vi "GV_Bypass_Main.vi"() -> ()   [LabVIEW 2019]
uses:
  GV_Bypass_Global.vi
panel:
  out "V0":dbl
  out "Status Code":i32 format="%x"
  in  "set_m001":bool
  in  "set_p001":bool
  in  "pressure_preset":T1(ring) caption="Presets"
  out "move_pre":i32 caption="Prev. move"
  out "status_ac":u32(colorbox) caption="Status"
  out "P_now":dbl caption="Fridge pressure" format="%.2f"
  in  "P_set":dbl=10.0 caption="Set Point" format="%.2f"
  in  "enable_auto_ctrl":bool caption="Auto Control\nwith Pressure"
  in  "set_m010":bool
  in  "set_m005":bool
  in  "set_p010":bool
  in  "set_p005":bool
  out "turn_now":dbl=-0.0 caption="turns" format="%.3f"
  out "step_rel_pre":i32 caption="Prev. steps"
  out "step_corr":i32
  in  "backlash_corr":bool=TRUE caption="Backlash Correction"
  in  "calib_zero":bool
  out "step_new":i32 caption="steps"
  in  "do_full_open":bool
  in  "do_full_close":bool
  in  "sp_turn":dbl caption="Set point:" min=-0.1 max=0.3 step=0.001 format="%.3f"
  out "Status":bool=TRUE
  out "Chart":waveform(dbl)[](graph)=[{"t0"=timestamp(3783179446.718648 s since 1904-01-01), "dt"=1.0, "Y"=[-0.0], "attributes"=variant("NI_ChannelName"=variant(string "Turn"))}, {"t0"=timestamp(3783179446.718648 s since 1904-01-01), "dt"=1.0, "Y"=[0.0], "attributes"=variant("NI_ChannelName"=variant(string "Step"))}, {"t0"=timestamp(3783179446.718648 s since 1904-01-01), "dt"=1.0, "Y"=[1.298], "attributes"=variant("NI_ChannelName"=variant(string "Analog"))}]
  out "Last Measurement":timestamp=timestamp(3783179446.718648 s since 1904-01-01) format="%<%Y-%m-%d %H:%M:%S>T"
  in  "Interval":i32=1000
  out "Open":bool
  out "Close":bool
  in  "MotorStop":bool
  in  "MotorEN":bool
  out "Alarm Code":i32 format="%x"
  in  "Alarm Reset":bool
  out "Analog":dbl=1.298
  in  "CLOSE Steps":i32=100
  out "step_now":i32 caption="steps"
  in  "OPEN Steps":i32=100
  in  "VISA":refnum<visa-resource-name>="COM13"
  in  "OPEN":bool
  in  "CLOSE":bool
  in  "stop":bool
  # "Gate-Valve Bypass Control"
  # "Gear ratio = 1:32.\nAnalog range = ?...?."
  # "ms"
  # "Absolute Moves"
  # "±0.001"
  # "turns"
  # "Present Position"
  # "Limit Switches"
  # "Relative Moves (Expert Only)"
  # "Torr"
  # "Fully Closed   = 0      turns =         0 steps\nFully Opened = 0.25 turns = -1600 steps"
  # "Torr"
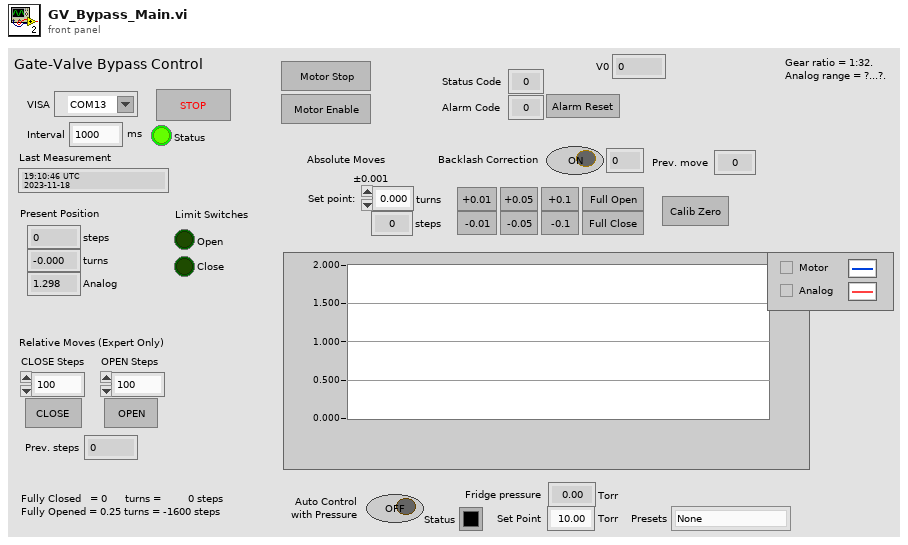
[diagram p1: front panel]
types:
  T1 = enum16{"None", "8.46 Torr  ->  1.7 K", "23.48 Torr  ->  2.0 K", "76.73 Torr  ->  2.5 K", "180.40 Torr  ->  3.0 K"}
  T2 = enum16{"None", "8.5 Torr  ->  1.7 K", "23.5 Torr  ->  2.0 K", "76.7 Torr  ->  2.5 K", "180.4 Torr  ->  3.0 K", ""}
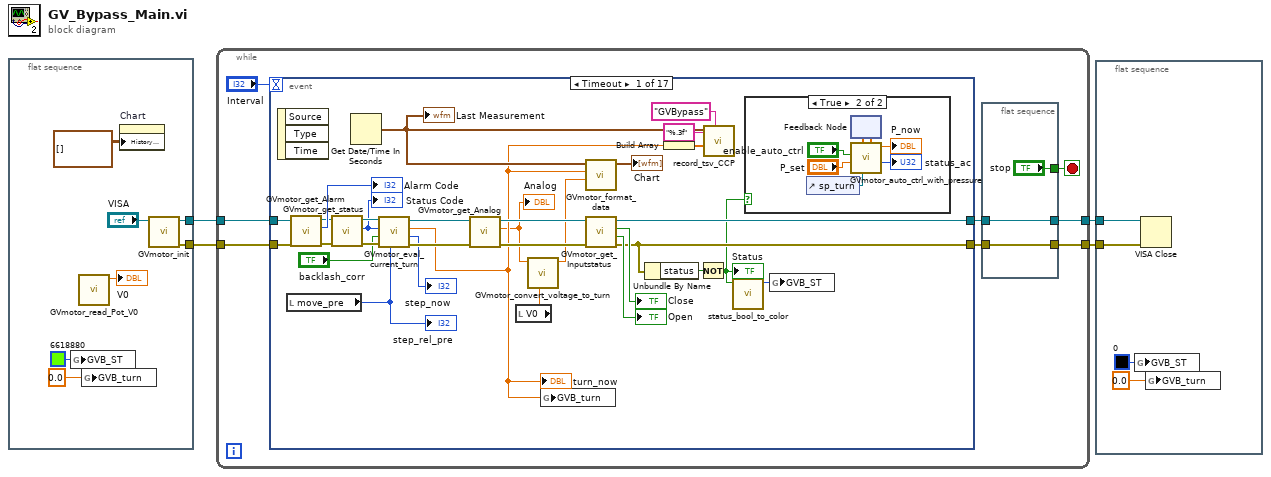
[diagram p0: block diagram]
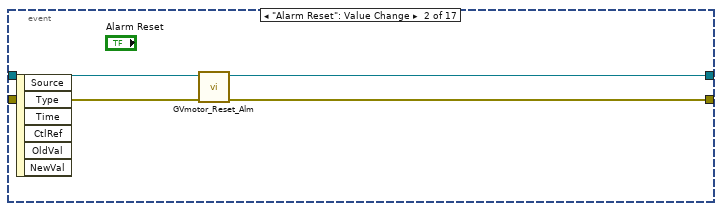
[diagram p3: hidden frame]
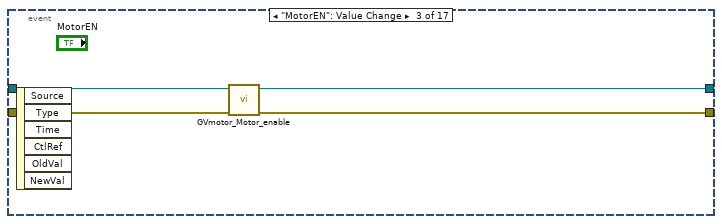
[diagram p4: hidden frame]
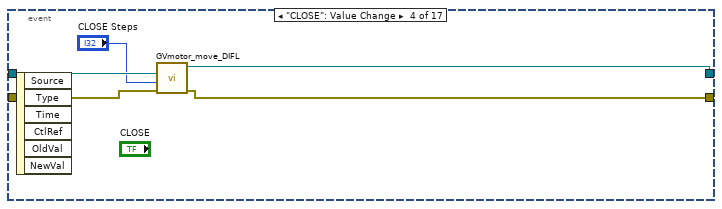
[diagram p5: hidden frame]
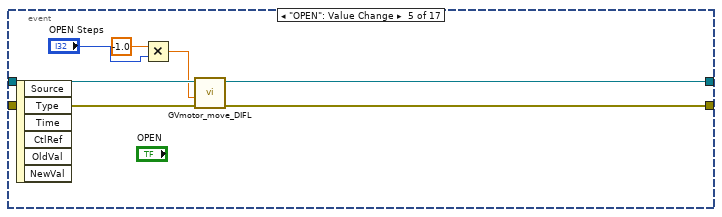
[diagram p6: hidden frame]
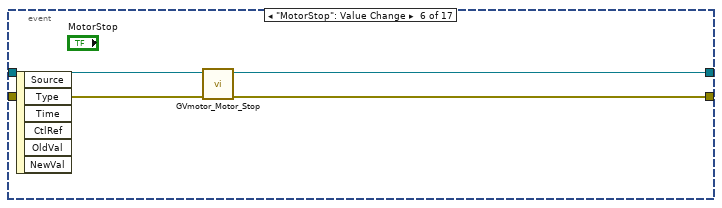
[diagram p7: hidden frame]
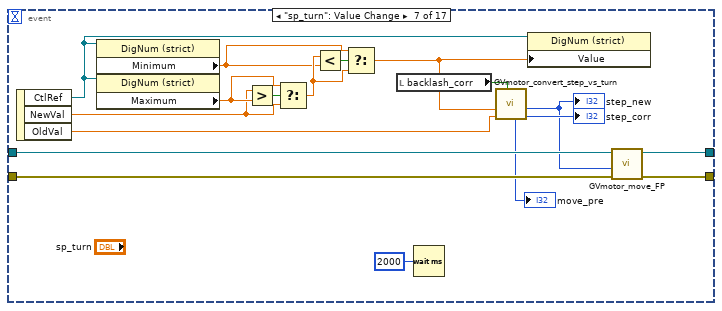
[diagram p8: hidden frame]
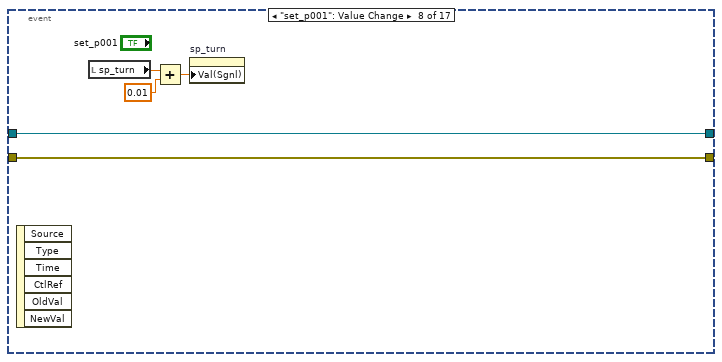
[diagram p9: hidden frame]
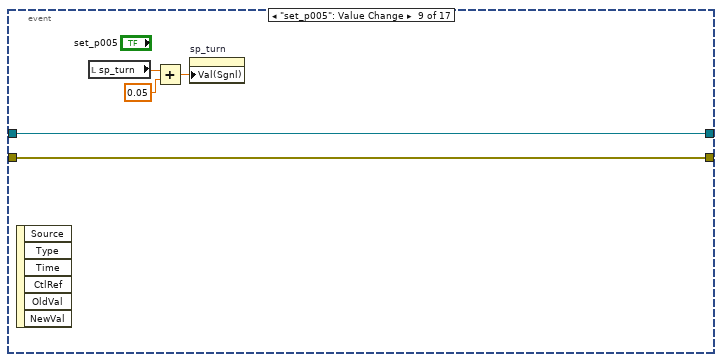
[diagram p10: hidden frame]
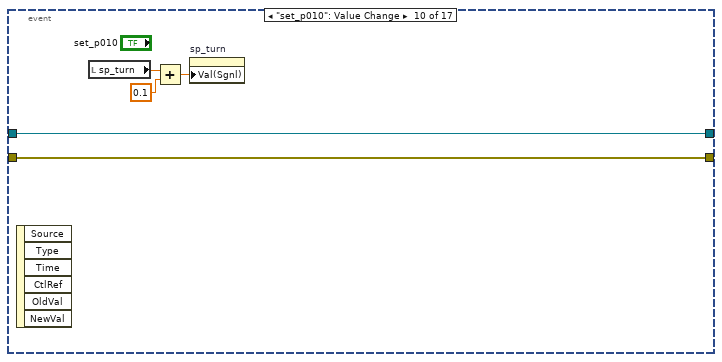
[diagram p11: hidden frame]
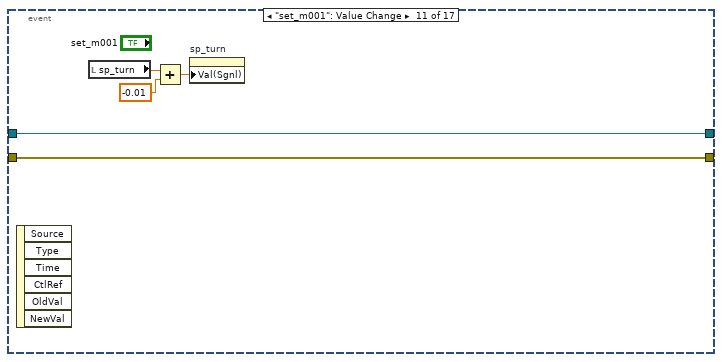
[diagram p12: hidden frame]
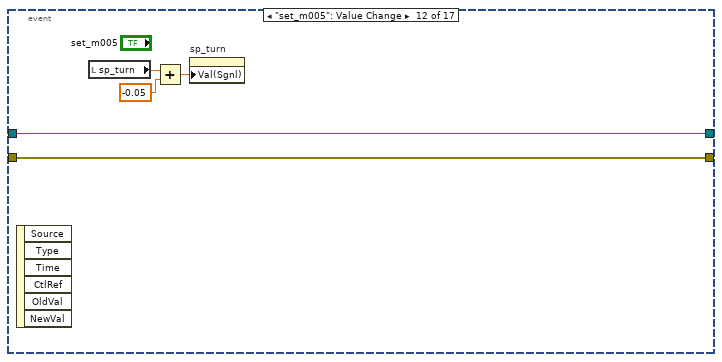
[diagram p13: hidden frame]
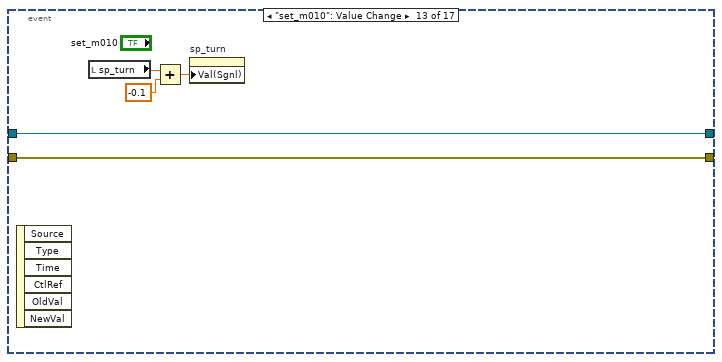
[diagram p14: hidden frame]
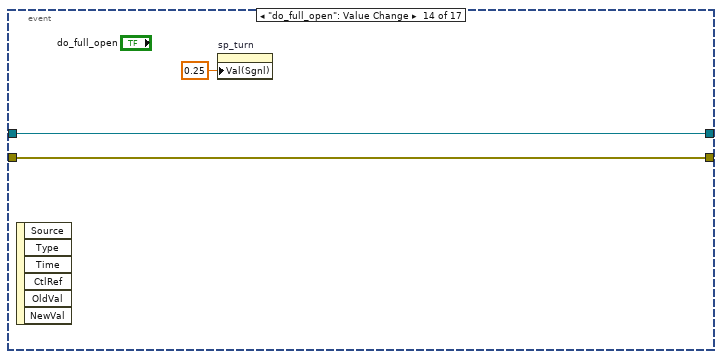
[diagram p15: hidden frame]
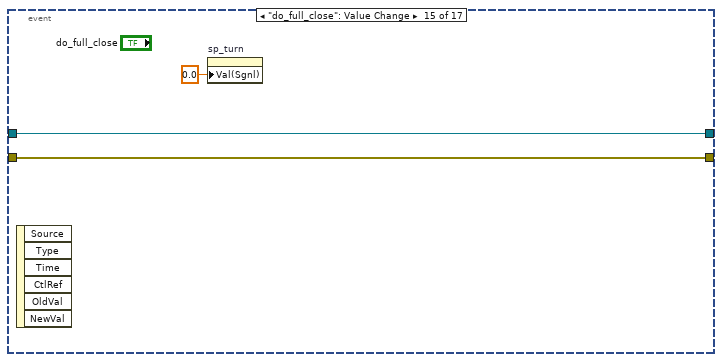
[diagram p16: hidden frame]
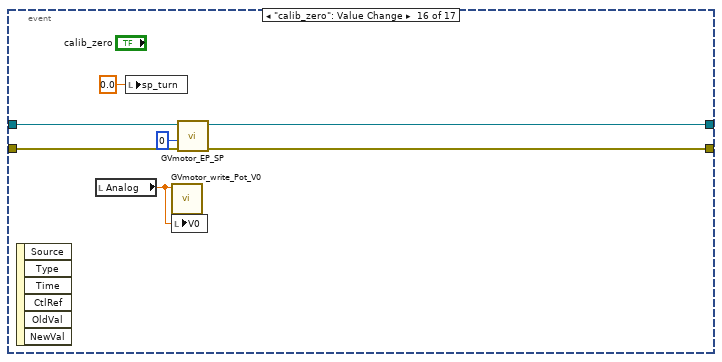
[diagram p17: hidden frame]
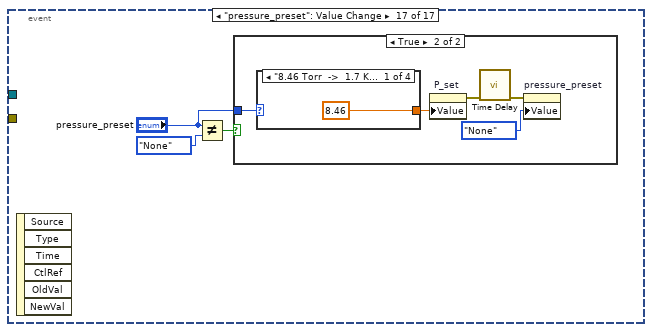
[diagram p18: hidden frame]
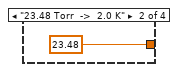
[diagram p20: hidden frame]
diagram:
  n1 = flat-sequence {
    tunnel: [w10] -> w4
    tunnel: [w9] -> w3
    frame #0 {
      n2 = global write "GV_Bypass_Global.vi" "GVB_ST"(u32 6618880 ("GVB_ST")) -> ()
      n3 = call "GVmotor_read_Pot_V0.vi"() -> ("V0"=→"V0":dbl)  [unwired: 11 in]
      n4 = global write "GV_Bypass_Global.vi" "GVB_turn"(0.0 ("GVB_opening")) -> ()
      n5 = property on="Chart" class="WFChart (strict)"("History Data"=waveform(dbl)[][] []) -> ()  [unwired: 2 in, 2 out]
      n6 = call "GVmotor_init.vi"("mWMotor_Port"="VISA") -> ("error out"=w9:errorcluster, "reference out"=w10:refnum<visa-resource-name>)  [unwired: 9 in]
    }
  }
  n7 = while {
    tunnel: w4 -> [w17]
    tunnel: w3 -> [w16]
    tunnel: [w12] -> w2
    tunnel: [w14] -> w1
    stop <- w19 stop-if-true
    n8 = event shown="[0] Timeout" {
      selector: _ -> [_ _ _ _ _ _ _ _ _ _ _ _ _ _ _ _ _]
      dyn-events: _ -> [_ _ _ _ _ _ _ _ _ _ _ _ _ _ _ _ _]
      timeout: "Interval" -> [_ _ _ _ _ _ _ _ _ _ _ _ _ _ _ _ _]
      tunnel: w17 -> [w37 w62 w65 w73 w80 w81 w87 w107 w112 w117 w122 w127 w132 w134 w137 w145 _]
      tunnel: w16 -> [w36 w63 w68 w72 w79 w84 w88 w106 w111 w116 w121 w126 w131 w133 w136 w143 _]
      tunnel: [w45 w64 w67 w71 w78 w83 w89 w106 w111 w116 w121 w126 w131 w133 w136 w142 _] -> w13
      tunnel: [w46 w61 w66 w70 w77 w82 w90 w107 w112 w117 w122 w127 w132 w134 w137 w144 _] -> w15
      event Timeout {
        n9 = event-data() -> ()  [unwired: 1 in, 3 out]
        n10 = local read "move_pre"() -> (w27:i32)
        "step_rel_pre" <- w27
        n11 = call "GVmotor_get_Alarm.vi"("error in (no error)"=w36, "VISA resource name"=w37) -> ("error out"=w35:errorcluster, "Alarm Code"=→"Alarm Code":i32, "VISA resource name out"=w34:refnum<visa-resource-name>)  [unwired: 7 in]
        n12 = call "GVmotor_get_status.vi"("error in"=w35, "VISA in"=w34) -> ("error out"=w32:errorcluster, "Status Code"=w29:i32, "VISA out"=w33:refnum<visa-resource-name>)  [unwired: 7 in]
        "Status Code" <- w29
        n13 = Get Date/Time In Seconds() -> (seconds since 1Jan1904=w42:timestamp)
        "Last Measurement" <- w42
        n14 = call "GVmotor_eval_current_turn.vi"("move_pre_sign"=w27, "error in"=w32, "backlash_corr"="backlash_corr", "status_code"=w29, "VISA in"=w33) -> ("error out"=w47:errorcluster, "step_curr"=→"step_now":i32, "turn_curr"=w26:dbl, "VISA out"=w48:refnum<visa-resource-name>)  [unwired: 3 in]
        "turn_now" <- w26
        n15 = call "GVmotor_get_Analog.vi"("error in (no error)"=w47, "VISA resource name"=w48) -> ("error out"=w30:errorcluster, "Analog"=w25:dbl, "VISA resource name out"=w31:refnum<visa-resource-name>)  [unwired: 7 in]
        "Analog" <- w25
        n16 = local read "V0"() -> (w23:dbl)
        n17 = call "GVmotor_convert_voltage_to_turn.vi"("v0"=w23, "voltage"=w25) -> ("turn"=w24:dbl)  [unwired: 8 in, 1 out]
        n18 = global write "GV_Bypass_Global.vi" "GVB_turn"(w26) -> ()
        n19 = call "GVmotor_format_data.vi"("analog"=w24, "turn"=w26, "time"=w42) -> ("waveform_array"=→"Chart":waveform(dbl)[])  [unwired: 8 in]
        n20 = call "GVmotor_get_Inputstatus.vi"("error in (no error)"=w30, "VISA resource name"=w31) -> ("error out"=w45:errorcluster, "Open"=→"Open":bool, "Close"=→"Close":bool, "VISA resource name out"=w46:refnum<visa-resource-name>)  [unwired: 6 in]
        n21 = Unbundle By Name(w45) -> ("status"=w50:bool)
        n22 = Build Array(w26) -> (w43:dbl[])
        n23 = Not(x=w50) -> (.not. x?=w39:bool)
        "Status" <- w39
        n24 = call "record_tsv_CCP.vi"("folder_name"="GVBypass", "value_array"=w43, "format"="%.3f", "time"=w42) -> ()  [unwired: 6 in, 2 out]
        n25 = call "status_bool_to_color.vi"("status_bool_1"=w39) -> ("status_color"=w49:u32)  [unwired: 10 in]
        n26 = case shown="True" w39 {
          frame False {
          }
          frame True {
            n27 = control-ref of="sp_turn"() -> (w54:refnum<vi>)
            n28 = feedback #1() -> (w59:dbl[])  [unwired: 1 in]
            n29 = call "GVmotor_auto_ctrl_with_pressure.vi"("ref_turn_set"=w54, "array_value_in"=w59, "P_set"="P_set", "enable_auto_ctrl"="enable_auto_ctrl") -> ("auto_ctrl_status"=→"status_ac":u32, "P_now"=→"P_now":dbl, "array_value_out"=w60:dbl[])  [unwired: 4 in, 1 out]
            n30 = feedback-in #1(w60) -> ()
          }
        }
        n31 = global write "GV_Bypass_Global.vi" "GVB_ST"(w49) -> ()
      }
      event "Alarm Reset": Value Change {
        n32 = event-data() -> ()  [unwired: 1 in, 6 out]
        n33 = call "GVmotor_Reset_Alm.vi"("error in (no error)"=w63, "VISA resource name"=w62) -> ("error out"=w64:errorcluster, "VISA resource name out"=w61:refnum<visa-resource-name>)  [unwired: 8 in]
      }
      event "MotorEN": Value Change {
        n34 = event-data() -> ()  [unwired: 1 in, 6 out]
        n35 = call "GVmotor_Motor_enable.vi"("error in (no error)"=w68, "VISA resource name"=w65) -> ("error out"=w67:errorcluster, "VISA resource name out"=w66:refnum<visa-resource-name>)  [unwired: 8 in]
      }
      event "CLOSE": Value Change {
        n36 = event-data() -> ()  [unwired: 1 in, 6 out]
        n37 = call "GVmotor_move_DIFL.vi"("error in"=w72, "relative_step"="CLOSE Steps", "VISA in"=w73) -> ("error out"=w71:errorcluster, "VISA out"=w70:refnum<visa-resource-name>)  [unwired: 7 in]
      }
      event "OPEN": Value Change {
        n38 = event-data() -> ()  [unwired: 1 in, 6 out]
        n39 = Multiply(x=-1.0, y="OPEN Steps") -> (x*y=w76:dbl)
        n40 = call "GVmotor_move_DIFL.vi"("error in"=w79, "relative_step"=w76, "VISA in"=w80) -> ("error out"=w78:errorcluster, "VISA out"=w77:refnum<visa-resource-name>)  [unwired: 7 in]
      }
      event "MotorStop": Value Change {
        n41 = event-data() -> ()  [unwired: 1 in, 6 out]
        n42 = call "GVmotor_Motor_Stop.vi"("error in (no error)"=w84, "VISA resource name"=w81) -> ("error out"=w83:errorcluster, "VISA resource name out"=w82:refnum<visa-resource-name>)  [unwired: 8 in]
      }
      event "sp_turn": Value Change {
        n43 = event-data() -> ("CtlRef"=w91:refnum<vi>, "NewVal"=w93:dbl, "OldVal"=w102:dbl)  [unwired: 1 in]
        n44 = property class="DigNum (strict)"(reference=w91) -> ("Minimum"=w95:dbl)  [unwired: 1 in, 2 out]
        n45 = property class="DigNum (strict)"(reference=w91) -> ("Maximum"=w94:dbl)  [unwired: 1 in, 2 out]
        n46 = Greater?(x=w93, y=w94) -> (0:w98:bool)
        n47 = Select(t=w94, s=w98, f=w93) -> (s? t:f=w96:dbl)
        n48 = Less?(x=w96, y=w95) -> (x < y?=w97:bool)
        n49 = Select(t=w95, s=w97, f=w96) -> (s? t:f=w92:dbl)
        n50 = local read "backlash_corr"() -> (w100:bool)
        n51 = Wait (ms)(milliseconds to wait=u32 2000) -> ()  [unwired: 1 out]
        n52 = call "GVmotor_convert_step_vs_turn.vi"("backlash_corr"=w100, "turn_in_pre"=w102, "turn_in"=w92) -> ("step_corr_for_step_out"=→"step_corr":i32, "step_out"=w86:i32, "step_change_sign"=→"move_pre":i8)  [unwired: 4 in, 2 out]
        "step_new" <- w86
        n53 = property class="DigNum (strict)"(reference=w91, "Value"=w92) -> ()  [unwired: 1 in, 2 out]
        n54 = call "GVmotor_move_FP.vi"("error in"=w88, "Steps"=w86, "VISA in"=w87) -> ("error out"=w89:errorcluster, "VISA out"=w90:refnum<visa-resource-name>)  [unwired: 7 in]
      }
      event "set_p001": Value Change {
        n55 = event-data() -> ()  [unwired: 1 in, 6 out]
        n56 = local read "sp_turn"() -> (w105:dbl)
        n57 = Add(x=w105, y=0.01) -> (x+y=w104:dbl)
        n58 = property on="sp_turn" class="DigNum (strict)"("Val(Sgnl)"=w104) -> ()  [unwired: 2 in, 2 out]
      }
      event "set_p005": Value Change {
        n59 = event-data() -> ()  [unwired: 1 in, 6 out]
        n60 = local read "sp_turn"() -> (w110:dbl)
        n61 = Add(x=w110, y=0.05) -> (x+y=w109:dbl)
        n62 = property on="sp_turn" class="DigNum (strict)"("Val(Sgnl)"=w109) -> ()  [unwired: 2 in, 2 out]
      }
      event "set_p010": Value Change {
        n63 = event-data() -> ()  [unwired: 1 in, 6 out]
        n64 = local read "sp_turn"() -> (w115:dbl)
        n65 = Add(x=w115, y=0.1) -> (x+y=w114:dbl)
        n66 = property on="sp_turn" class="DigNum (strict)"("Val(Sgnl)"=w114) -> ()  [unwired: 2 in, 2 out]
      }
      event "set_m001": Value Change {
        n67 = event-data() -> ()  [unwired: 1 in, 6 out]
        n68 = local read "sp_turn"() -> (w120:dbl)
        n69 = Add(x=w120, y=-0.01) -> (x+y=w119:dbl)
        n70 = property on="sp_turn" class="DigNum (strict)"("Val(Sgnl)"=w119) -> ()  [unwired: 2 in, 2 out]
      }
      event "set_m005": Value Change {
        n71 = event-data() -> ()  [unwired: 1 in, 6 out]
        n72 = local read "sp_turn"() -> (w125:dbl)
        n73 = Add(x=w125, y=-0.05) -> (x+y=w124:dbl)
        n74 = property on="sp_turn" class="DigNum (strict)"("Val(Sgnl)"=w124) -> ()  [unwired: 2 in, 2 out]
      }
      event "set_m010": Value Change {
        n75 = event-data() -> ()  [unwired: 1 in, 6 out]
        n76 = local read "sp_turn"() -> (w130:dbl)
        n77 = Add(x=w130, y=-0.1) -> (x+y=w129:dbl)
        n78 = property on="sp_turn" class="DigNum (strict)"("Val(Sgnl)"=w129) -> ()  [unwired: 2 in, 2 out]
      }
      event "do_full_open": Value Change {
        n79 = event-data() -> ()  [unwired: 1 in, 6 out]
        n80 = property on="sp_turn" class="DigNum (strict)"("Val(Sgnl)"=0.25 ("Value (Signaling)")) -> ()  [unwired: 2 in, 2 out]
      }
      event "do_full_close": Value Change {
        n81 = event-data() -> ()  [unwired: 1 in, 6 out]
        n82 = property on="sp_turn" class="DigNum (strict)"("Val(Sgnl)"=0.0 ("Value (Signaling)")) -> ()  [unwired: 2 in, 2 out]
      }
      event "calib_zero": Value Change {
        n83 = event-data() -> ()  [unwired: 1 in, 6 out]
        n84 = local read "Analog"() -> (w139:dbl)
        n85 = local write "sp_turn"(0.0 ("sp_turn")) -> ()
        n86 = call "GVmotor_write_Pot_V0.vi"("V0"=w139) -> ()  [unwired: 11 in]
        n87 = local write "V0"(w139) -> ()
        n88 = call "GVmotor_EP_SP.vi"("error in"=w143, "pos"=0, "VISA in"=w145) -> ("error out"=w142:errorcluster, "VISA out"=w144:refnum<visa-resource-name>)  [unwired: 7 in]
      }
      event "pressure_preset": Value Change {
        n89 = event-data() -> ()  [unwired: 1 in, 6 out]
        n90 = Not Equal?(x="pressure_preset", y=T2."None") -> (x != y?=w147:bool)
        n91 = case shown="True" w147 {
          tunnel: "pressure_preset" -> [_ w153]
          frame False {
          }
          frame True {
            n92 = case shown="\"8.46 Torr  ->  1.7 K\", Default" w153 {
              tunnel: [8.46 23.48 76.73 180.4] -> w152
              frame "8.46 Torr  ->  1.7 K", Default {
              }
              frame "23.48 Torr  ->  2.0 K" {
              }
              frame "76.73 Torr  ->  2.5 K" {
              }
              frame "180.40 Torr  ->  3.0 K" {
              }
            }
            n93 = property on="P_set" class="DigNum (strict)"("Value"=w152) -> (error out=w151:errorcluster)  [unwired: 2 in, 1 out]
            n94 = call "Time Delay"("error in (no error)"=w151) -> ("error out"=w150:errorcluster)  [unwired: 10 in]
            n95 = property on="pressure_preset" class="Enum (strict)"(error in=w150, "Value"=T1."None" ("pressure_preset")) -> ()  [unwired: 1 in, 2 out]
          }
        }
      }
    }
    n96 = flat-sequence {
      tunnel: ["stop"] -> w19
      tunnel: w15 -> [w21]
      tunnel: [w21] -> w14
      tunnel: w13 -> [w20]
      tunnel: [w20] -> w12
      frame #0 {
      }
    }
  }
  n97 = flat-sequence {
    tunnel: w2 -> [w161]
    tunnel: w1 -> [w160]
    frame #0 {
      n98 = global write "GV_Bypass_Global.vi" "GVB_ST"(u32 0 ("GVB_ST")) -> ()
      n99 = VISA Close(VISA resource name=w160, error in (no error)=w161) -> ()  [unwired: 1 out]
      n100 = global write "GV_Bypass_Global.vi" "GVB_turn"(0.0 ("GVB_opening")) -> ()
    }
  }
